vi "Gerador de numeros inteiros entre 1 e 100.vi"() -> (0 "Numeric":dbl)   [LabVIEW 2018]
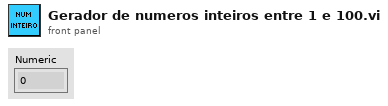
[diagram p1: front panel]
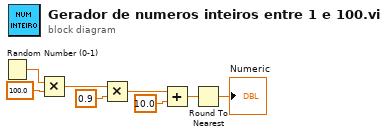
[diagram p0: block diagram]
diagram:
  n1 = Random Number (0-1)() -> (number: 0 to 1=w7:dbl)
  n2 = Multiply(x=w7, y=100.0) -> (x*y=w4:dbl)
  n3 = Multiply(x=w4, y=0.9) -> (x*y=w3:dbl)
  n4 = Add(x=w3, y=10.0) -> (x+y=w2:dbl)
  n5 = Round To Nearest(number=w2) -> (nearest integer value=→"Numeric":dbl)
